vi "Config FX Set.vi"(5 "Max # Of Tries":i32, 6 "Send Cmd Timout(ms)":u32=300, 8 "Error":errorcluster, 9 "HW Config":T6={"LiftHW Ver"=0, "CAN"={"ID Primary"=0, "Bus"="", "ID Follower"=0}, "Output"={"Type"=enum."Counter-Clockwise", "Neutral"=enum."EEPROMSetting", "Max"={"FWD"=0.0, "REV"=-1.0}, "Min"={"FWD"=0.0, "REV"=0.0}, "OL Ramp Rate (S)"=0.0, "Dead Band"=0.0}, "CLUp"={"Gains"={"P"=1.0, "I"=0.01, "D"=0.0, "F"=0.0}, "Error Allowed"={"High"=0.0, "Low"=0.0}, "I Zone"={"High"=10000.0, "Low"=-1000.0}, "Max Out"={"FWD"=1.0, "REV"=-1.0}, "Max I Accu"={"High"=10.0, "Low"=-10.0}, "CL Ramp Rate (S)"=0.0}, "MM"={"Cruise Velocity"=5000, "Acceleration"=5000}, "TravelLimits"={"Hard"={"FWD Switch Normal"=enum."Normally Open", "FWD On will Zero Encoder "=FALSE, "REV Switch Normal"=enum."Normally Open", "REV On will Zero Encoder "=FALSE}, "Soft"={"FWD"={"Enable"=FALSE, "Counts"=0}, "REV"={"Enable"=FALSE, "Counts"=0}}}, "Cancoder"={"ID"=0, "CW(t) CCW(f)"=TRUE, "Zero Offset"=0.0}, "CLDown"={"Gains"={"P"=1.0, "I"=0.01, "D"=0.0, "F"=0.0}, "Error Allowed"={"High"=0.0, "Low"=0.0}, "I Zone"={"High"=10000.0, "Low"=-1000.0}, "Max Out"={"FWD"=1.0, "REV"=-1.0}, "Max I Accu"={"High"=10.0, "Low"=-10.0}, "CL Ramp Rate (S)"=0.0}, "CurrentLimit"={"Enable"=FALSE, "Current Limit"=0.0, "Threshold Current"=0.0, "Threshold Time"=0.0}} {"CLDown"."Max I Accu"."Low" format="%#.8f"; "CLDown"."Max I Accu"."High" format="%#.8f"; "CLDown"."Gains"."F" format="%#.8f"; "CLDown"."Gains"."D" format="%#.8f"; "CLDown"."Gains"."I" format="%#.8f"; "CLDown"."Gains"."P" format="%#.8f"; "CLDown"."Error Allowed"."Low" format="%#.8f"; "CLDown"."Error Allowed"."High" format="%#.8f"; "CLDown"."I Zone"."Low" format="%#.8f"; "CLDown"."I Zone"."High" format="%#.8f"; "CLDown"."Max Out"."REV" format="%.2f"; "CLDown"."Max Out"."FWD" format="%.2f"; "TravelLimits"."Soft"."REV"."Counts" format="%#.0f"; "TravelLimits"."Soft"."FWD"."Counts" format="%#.0f"; "Output"."Min"."REV" format="%.2f"; "Output"."Min"."FWD" format="%.2f"; "Output"."Max"."REV" format="%.2f"; "Output"."Max"."FWD" format="%.2f"; "CLUp"."Max I Accu"."Low" format="%#.8f"; "CLUp"."Max I Accu"."High" format="%#.8f"; "CLUp"."Gains"."F" format="%#.8f"; "CLUp"."Gains"."D" format="%#.8f"; "CLUp"."Gains"."I" format="%#.8f"; "CLUp"."Gains"."P" format="%#.8f"; "CLUp"."Error Allowed"."Low" format="%#.8f"; "CLUp"."Error Allowed"."High" format="%#.8f"; "CLUp"."I Zone"."Low" format="%#.8f"; "CLUp"."I Zone"."High" format="%#.8f"; "CLUp"."Max Out"."REV" format="%.2f"; "CLUp"."Max Out"."FWD" format="%.2f"}, 11 "PhoenixMotorControlDevRef":T1={"DeviceStatus"={"status"=FALSE, "code"=0, "source"=""}, "Type"=enum."PWM", "PWM"={"PWM Channel"=enum."Invalid", "DeadBand"={"Name"="", "maxPositivePwm"=0, "minPositivePwm"=0, "centerPwm"=0, "maxNegativePwm"=0, "minNegativePwm"=0, "angularRange"=0}}, "CAN"={"Device Number"=0, "SetOutput VI Ref"=variant, "GetOutput VI Ref"=variant, "Enable VI Ref"=variant, "Disable VI Ref"=variant, "Data"=variant}, "Invert"=FALSE, "DIO PWM"={"PWM \"Enable\" Channel"=enum."Invalid", "DIOChannel"=enum."Invalid", "PWM Rate"=0.0}}) -> (0 "Error Out":errorcluster, 3 "PhoenixMotorControlDevRef Out Out":T1)   [LabVIEW 2023, in "Lift_ACT.lvlib"]
uses:
  Lift_ACT.lvlib
  <vilib>/Utility/Data Type/NI_Data Type.lvlib
  Shared Code/TypeDefs/Cluser_CAN Data.ctl
  <vilib>/Rock Robotics/WPI/ThirdParty/Phoenix-LabVIEW/Motor Controller/Controls/CTRE_Phoenix_MotorControl_TalonFXInvertType.ctl
  <vilib>/Rock Robotics/WPI/ThirdParty/Phoenix-LabVIEW/Motor Controller/Controls/CTRE_Phoenix_MotorControl_NeutralMode.ctl
  Shared Code/TypeDefs/Cluster_FWD  REV Values.ctl
  Shared Code/TypeDefs/Cluster_Config Motor Output.ctl
  Shared Code/TypeDefs/Cluster_PID Gains.ctl
  Shared Code/TypeDefs/Cluster_High-Low.ctl
  Shared Code/TypeDefs/Cluster_PID Config.ctl
  Shared Code/TypeDefs/Cluster_Motion Magic Parameters.ctl
  <vilib>/Rock Robotics/WPI/ThirdParty/Phoenix-LabVIEW/Motor Controller/Controls/CTRE_Phoenix_MotorControl_LimitSwitchNormal.ctl
  Shared Code/TypeDefs/Cluser_Hard Limits.ctl
  Shared Code/TypeDefs/Cluser_Enable-Value I32.ctl
  Shared Code/TypeDefs/Cluser_Config_Soft Limits.ctl
  Shared Code/TypeDefs/Cluser_Limit Travel Config.ctl
  <vilib>/Rock Robotics/WPI/ThirdParty/Phoenix-LabVIEW/Motor Controller/Controls/CTRE_Phoenix_MotorControl_RemoteSourceType.ctl
  <vilib>/Rock Robotics/WPI/ThirdParty/Phoenix-LabVIEW/Motor Controller/Controls/CTRE_Phoenix_MotorControl_FeedbackDevice_TalonFX.ctl
  Shared Code/TypeDefs/Cluster_Config FX Motor Output.ctl
  Shared Code/TypeDefs/Cluster_FX SLOT PID Config.ctl
  <vilib>/Rock Robotics/SystemInterfaces/DIO/FPGA_DIOPWMChannel.ctl
  <vilib>/Rock Robotics/WPI/PWM/WPI_PWMDeadband.ctl
  <vilib>/Rock Robotics/WPI/MotorControl/WPI_MotorControlType.ctl
  <vilib>/Rock Robotics/SystemInterfaces/DIO/FPGA_DIOChannel.ctl
  <vilib>/Rock Robotics/WPI/MotorControl/WPI_MotorControlDeviceRef.ctl
  Shared Code/TypeDefs/Cluster_Config_Cancoder Data.ctl
  Shared Code/TypeDefs/Cluster_Lift_Config HW Values.ctl
  Shared Code/TypeDefs/Cluser_CAN Follower Data.ctl
  Shared Code/TypeDefs/Cluser_Config_Current Limits.ctl
panel:
  # "Tune Output\nto 1023 Max"
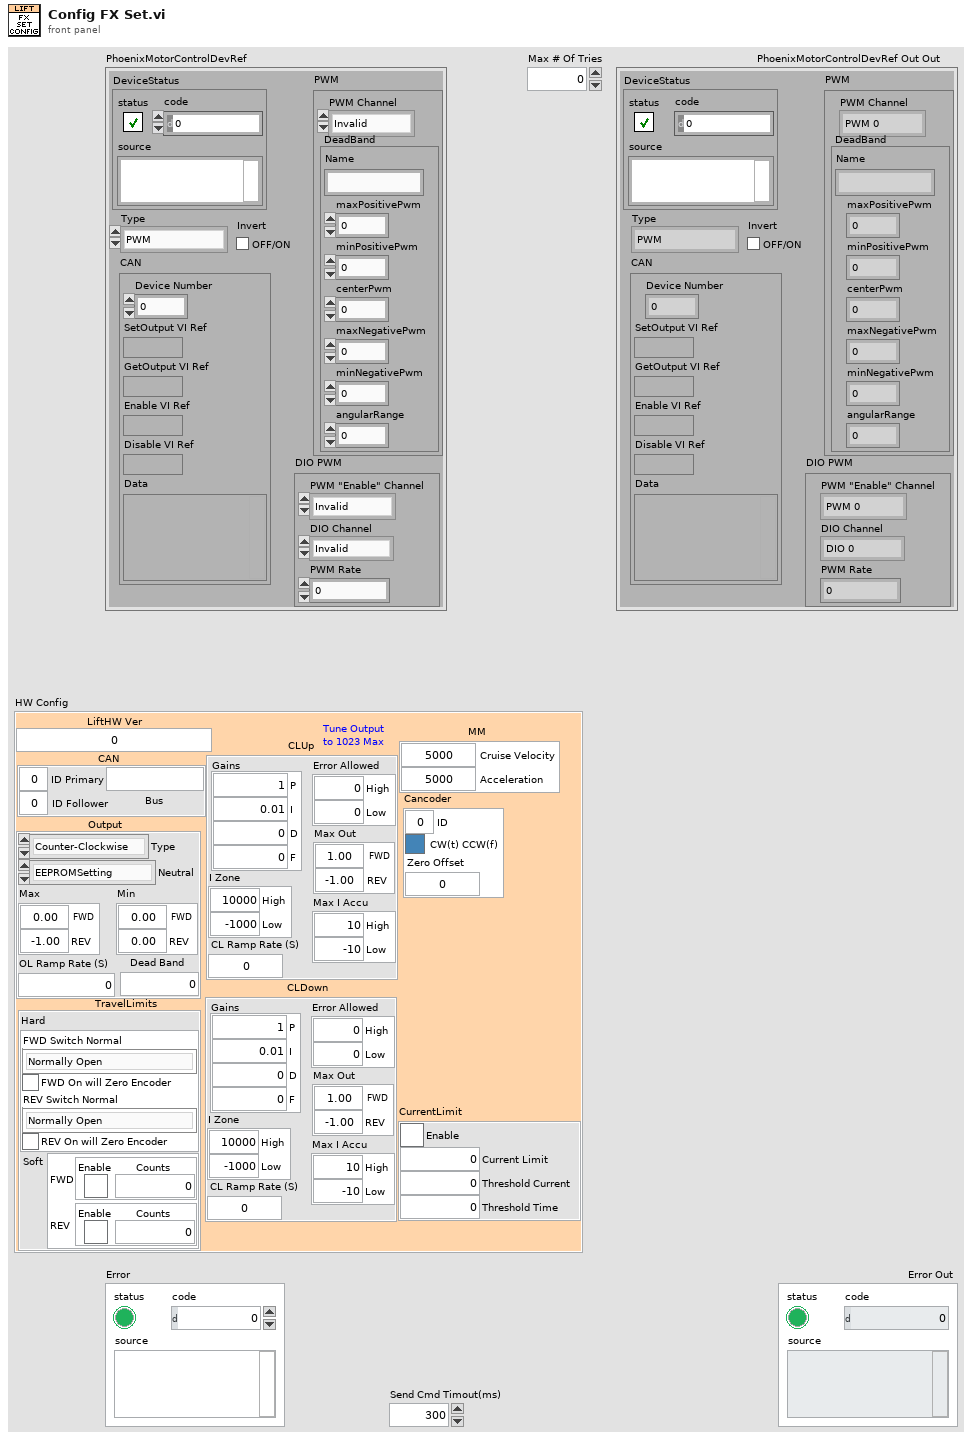
[diagram p1: front panel]
types:
  T1 = typedef "WPI_MotorControlDeviceRef.ctl" = cluster{"DeviceStatus":errorcluster, "Type":T2, "PWM":cluster{"PWM Channel":T3, "DeadBand":T4}, "CAN":cluster{"Device Number":u8, "SetOutput VI Ref":variant, "GetOutput VI Ref":variant, "Enable VI Ref":variant, "Disable VI Ref":variant, "Data":variant}, "Invert":bool, "DIO PWM":cluster{"PWM \"Enable\" Channel":T3, "DIOChannel":T5, "PWM Rate":dbl}}
  T2 = typedef "WPI_MotorControlType.ctl" = enum16{"PWM", "CAN", "DIO PWM"}
  T3 = typedef "FPGA_DIOPWMChannel.ctl" = enum8{"PWM 0", "PWM 1", "PWM 2", "PWM 3", "PWM 4", "PWM 5", "PWM 6", "PWM 7", "PWM 8", "PWM 9", "PWM MXP 0", "PWM MXP 1", "PWM MXP 2", "PWM MXP 3", "PWM MXP 4", "PWM MXP 5", "PWM MXP 6", "PWM MXP 7", "PWM MXP 8", "PWM MXP 9", "Invalid"}
  T4 = typedef "WPI_PWMDeadband.ctl" = cluster{"Name":string, "maxPositivePwm":i32, "minPositivePwm":i32, "centerPwm":i32, "maxNegativePwm":i32, "minNegativePwm":i32, "angularRange":u16}
  T5 = typedef "FPGA_DIOChannel.ctl" = enum8{"DIO 0", "DIO 1", "DIO 2", "DIO 3", "DIO 4", "DIO 5", "DIO 6", "DIO 7", "DIO 8", "DIO 9", "DIO MXP 0", "DIO MXP 1", "DIO MXP 2", "DIO MXP 3", "DIO MXP 4", "DIO MXP 5", "DIO MXP 6", "DIO MXP 7", "DIO MXP 8", "DIO MXP 9", "DIO MXP 10", "DIO MXP 11", "DIO MXP 12", "DIO MXP 13", "DIO MXP 14", "DIO MXP 15", "SPI Port CS1", "SPI Port CS2", "SPI Port CS3", "SPI Port MISO", "SPI Port MOSI", "Invalid"}
  T6 = typedef "Cluster_Lift_Config HW Values.ctl" = cluster{"LiftHW Ver":u64, "CAN":T7, "Output":T8, "CLUp":T12, "MM":T15, "TravelLimits":T16, "Cancoder":T21, "CLDown":T12, "CurrentLimit":T22}
  T7 = typedef "Cluser_CAN Follower Data.ctl" = cluster{"ID Primary":u8, "Bus":string, "ID Follower":u8}
  T8 = typedef "Cluster_Config Motor Output.ctl" = cluster{"Type":T9, "Neutral":T10, "Max":T11, "Min":T11, "OL Ramp Rate (S)":dbl, "Dead Band":dbl}
  T9 = typedef "CTRE_Phoenix_MotorControl_TalonFXInvertType.ctl" = enum16{"Counter-Clockwise", "Clockwise"}
  T10 = typedef "CTRE_Phoenix_MotorControl_NeutralMode.ctl" = enum8{"EEPROMSetting", "Override to Coast", "Override to Brake"}
  T11 = typedef "Cluster_FWD  REV Values.ctl" = cluster{"FWD":dbl, "REV":dbl}
  T12 = typedef "Cluster_PID Config.ctl" = cluster{"Gains":T13, "Error Allowed":T14, "I Zone":T14, "Max Out":T11, "Max I Accu":T14, "CL Ramp Rate (S)":dbl}
  T13 = typedef "Cluster_PID Gains.ctl" = cluster{"P":dbl, "I":dbl, "D":dbl, "F":dbl}
  T14 = typedef "Cluster_High-Low.ctl" = cluster{"High":dbl, "Low":dbl}
  T15 = typedef "Cluster_Motion Magic Parameters.ctl" = cluster{"Cruise Velocity":i32, "Acceleration":i32}
  T16 = typedef "Cluser_Limit Travel Config.ctl" = cluster{"Hard":T17, "Soft":T19}
  T17 = typedef "Cluser_Hard Limits.ctl" = cluster{"FWD Switch Normal":T18, "FWD On will Zero Encoder ":bool, "REV Switch Normal":T18, "REV On will Zero Encoder ":bool}
  T18 = typedef "CTRE_Phoenix_MotorControl_LimitSwitchNormal.ctl" = enum16{"Normally Open", "Normally Closed", "Disabled"}
  T19 = typedef "Cluser_Config_Soft Limits.ctl" = cluster{"FWD":T20, "REV":T20}
  T20 = typedef "Cluser_Enable-Value I32.ctl" = cluster{"Enable":bool, "Counts":i32}
  T21 = typedef "Cluster_Config_Cancoder Data.ctl" = cluster{"ID":u8, "CW(t) CCW(f)":bool, "Zero Offset":dbl}
  T22 = typedef "Cluser_Config_Current Limits.ctl" = cluster{"Enable":bool, "Current Limit":dbl, "Threshold Current":dbl, "Threshold Time":dbl}
  T23 = typedef "Cluser_CAN Data.ctl" = cluster{"ID":u8, "Bus":string}
  T24 = enum16{"FollowerType_PercentOutput", "FollowerType_AuxOutput1"}
  T25 = typedef "Cluster_FX SLOT PID Config.ctl" = cluster{"Gains":T13, "Error Allowed":dbl, "I Zone":dbl, "Peak Out 0-1":dbl, "Max I Accu":dbl}
  T26 = typedef "Cluster_Config FX Motor Output.ctl" = cluster{"Type":T9, "Neutral":T10, "Max":T11, "Min":T11, "OL Ramp Rate (S)":dbl, "Dead Band":dbl, "CL Ramp Rate (S)":dbl}
  T27 = typedef "CTRE_Phoenix_MotorControl_RemoteSourceType.ctl" = enum16{"Off", "Talon SRX Selected Sensor", "Pigeon IMU Yaw", "Pigeon IMU Pitch", "Pigeon IMU Roll", "CANifier Quadrature", "CANifier PWM Input 0", "CANifier PWM Input 1", "CANifier PWM Input 2", "CANifier PWM Input 3", "Gadgeteer Pigeon Yaw", "Gadgeteer Pigeon Pitch", "Gadgeteer Pigeon Roll", "CANCoder"}
  T28 = typedef "CTRE_Phoenix_MotorControl_FeedbackDevice_TalonFX.ctl" = i8
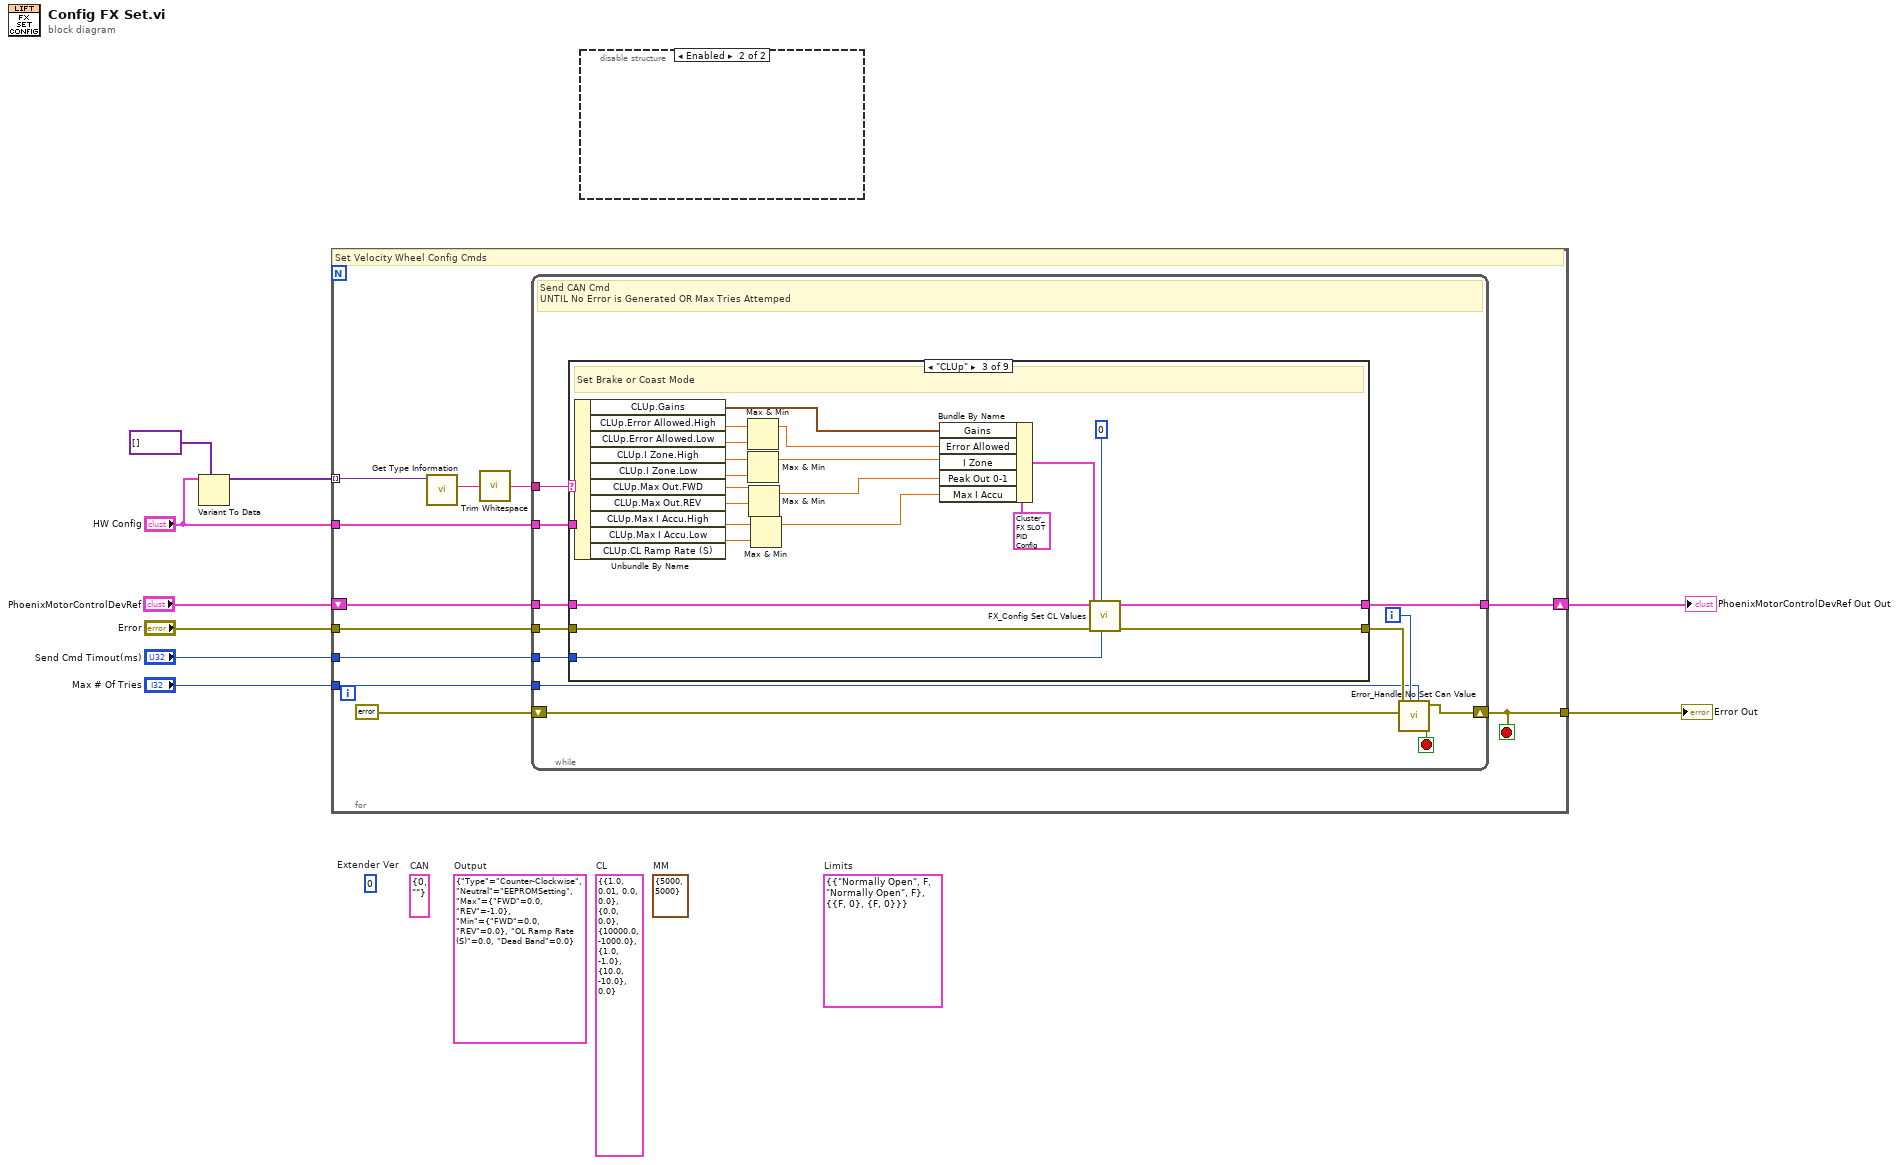
[diagram p0: block diagram]
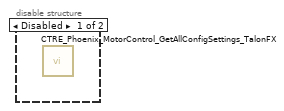
[diagram p2: hidden frame]
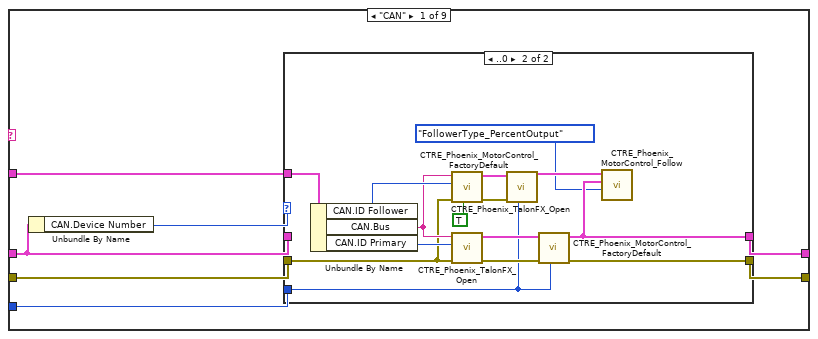
[diagram p3: hidden frame]
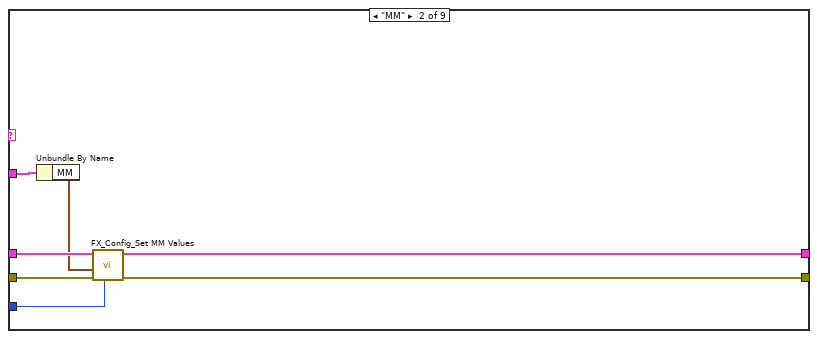
[diagram p5: hidden frame]
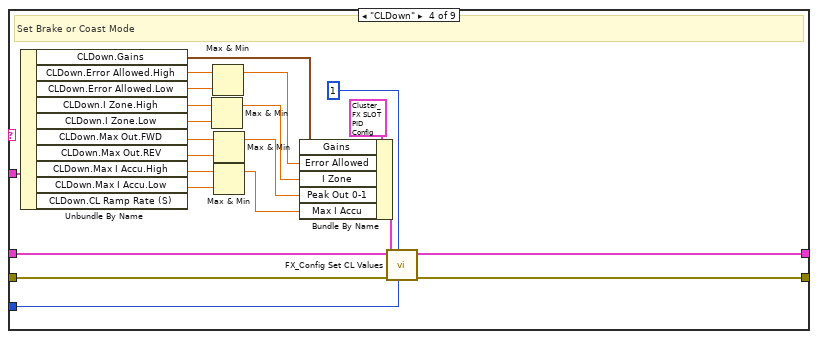
[diagram p6: hidden frame]
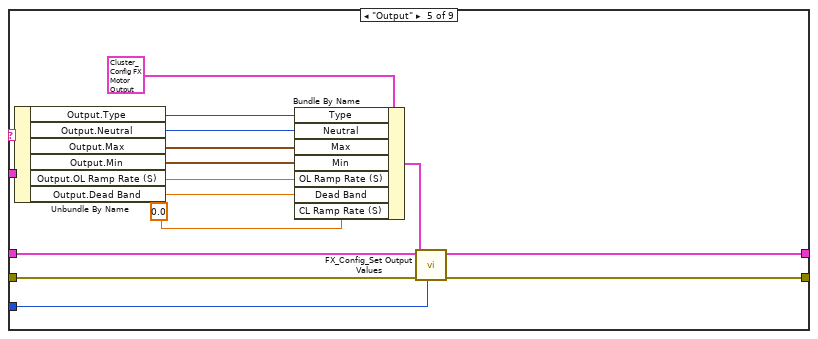
[diagram p7: hidden frame]
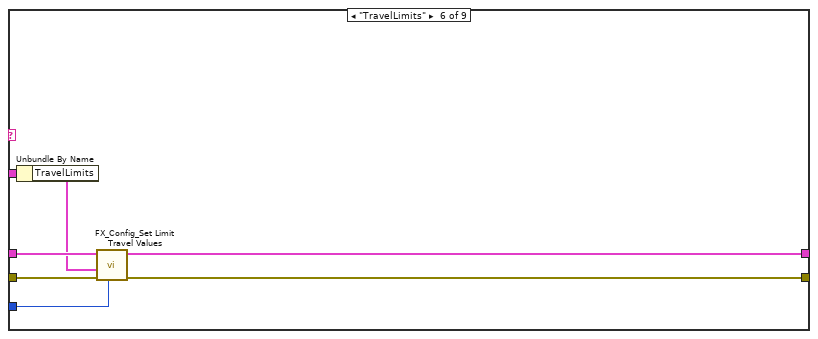
[diagram p8: hidden frame]
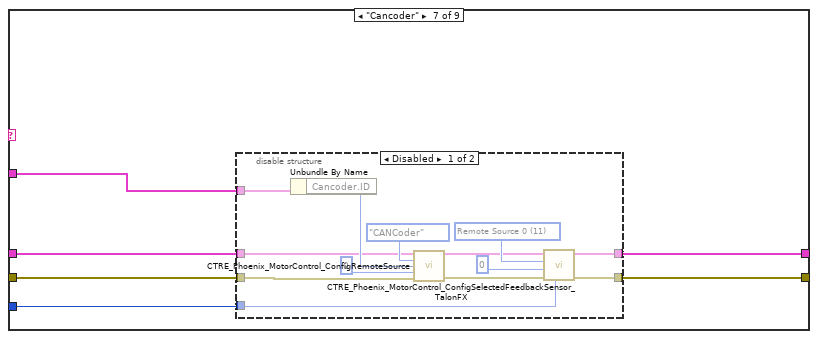
[diagram p9: hidden frame]
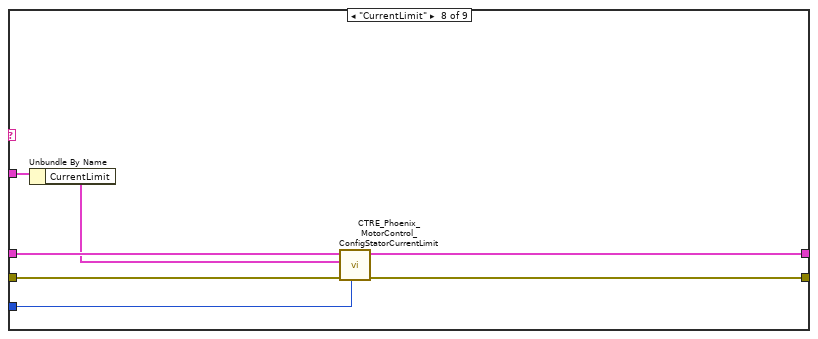
[diagram p11: hidden frame]
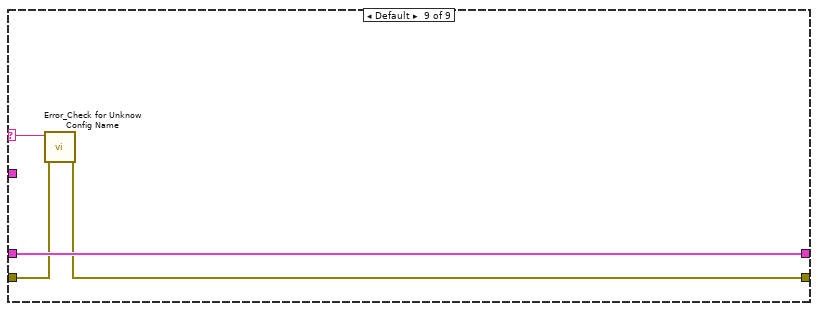
[diagram p12: hidden frame]
diagram:
  (unwired) T16 {"Hard"={"FWD Switch Normal"=enum."Normally Open", "FWD On will Zero Encoder "=FALSE, "REV Switch Normal"=enum."Normally Open", "REV On will Zero Encoder "=FALSE}, "Soft"={"FWD"={"Enable"=FALSE, "Counts"=0}, "REV"={"Enable"=FALSE, "Counts"=0}}}  # Limits
  (unwired) T15 {"Cruise Velocity"=5000, "Acceleration"=5000}  # MM
  (unwired) T12 {"Gains"={"P"=1.0, "I"=0.01, "D"=0.0, "F"=0.0}, "Error Allowed"={"High"=0.0, "Low"=0.0}, "I Zone"={"High"=10000.0, "Low"=-1000.0}, "Max Out"={"FWD"=1.0, "REV"=-1.0}, "Max I Accu"={"High"=10.0, "Low"=-10.0}, "CL Ramp Rate (S)"=0.0}  # CL
  (unwired) T8 {"Type"=enum."Counter-Clockwise", "Neutral"=enum."EEPROMSetting", "Max"={"FWD"=0.0, "REV"=-1.0}, "Min"={"FWD"=0.0, "REV"=0.0}, "OL Ramp Rate (S)"=0.0, "Dead Band"=0.0}  # Output
  (unwired) T23 {"ID"=0, "Bus"=""}  # CAN
  (unwired) u64 0  # Extender Ver
  n1 = Variant To Data(type=variant[] [] ("appended array"), Variant="HW Config") -> (data=w1:variant[])  [unwired: 1 in, 1 out]
  n2 = for {
    tunnel: "Send Cmd Timout(ms)" -> [w19]
    shift-right: [w20] -> w6
    shift-left: "PhoenixMotorControlDevRef" -> [w17]
    tunnel: "HW Config" -> [w18]
    tunnel: "Max # Of Tries" -> [w15]
    tunnel: w1 -> [w14] mode=indexing
    tunnel: "Error" -> [w16]
    tunnel: [w13] -> w5
    stop <- w13 stop-if-true
    # "Set Velocity Wheel Config Cmds"
    n3 = call <vilib>:"Get Type Information.vi"("variant"=w14) -> ("name"=w11:string)  [unwired: 6 in, 4 out]
    n4 = call <vilib>:"Trim Whitespace.vi"("string"=w11) -> ("trimmed string"=w10:string)  [unwired: 1 in]
    n5 = while {
      tunnel: [w24] -> w20
      tunnel: w19 -> [w30]
      shift-right: [w31] -> w13
      shift-left: errorcluster {"status"=FALSE, "code"=0, "source"=""} ("Error Out") -> [w29]
      tunnel: w16 -> [w27]
      tunnel: w17 -> [w26]
      tunnel: w18 -> [w25]
      tunnel: w15 -> [w23]
      tunnel: w10 -> [w22]
      i -> [w28]
      stop <- w21 stop-if-true
      # "Send CAN Cmd\nUNTIL No Error is Generated OR Max Tries Attemped"
      n6 = case shown="\"CLUp\"" w22 {
        selector: w22 -> [_ _ _ _ _ _ _ _ w160]
        tunnel: [w39 w62 w83 w105 w120 w127 w135 w157 w158] -> w32
        tunnel: w30 -> [w37 w61 w79 w101 w118 w125 w133 w155 _]
        tunnel: w27 -> [w38 w63 w82 w104 w119 w126 w134 w156 w159]
        tunnel: w26 -> [w35 w60 w85 w107 w121 w128 w132 w153 w161]
        tunnel: w25 -> [w33 w59 w81 w103 w117 w124 w130 w152 _]
        tunnel: [w34 w58 w84 w106 w122 w129 w131 w154 w161] -> w24
        frame "CAN" {
          n7 = Unbundle By Name(w35) -> ("CAN.Device Number"=w36:u8)
          n8 = case shown="..0" w36 {
            tunnel: [w40 w53] -> w39
            tunnel: w38 -> [w40 w46]
            tunnel: w37 -> [_ w49]
            tunnel: w35 -> [w41 _]
            tunnel: [w41 w44] -> w34
            tunnel: w33 -> [_ w52]
            frame 1.. {
            }
            frame ..0 {
              n9 = Unbundle By Name(w52) -> ("CAN.ID Follower"=w51:u8, "CAN.Bus"=w47:string, "CAN.ID Primary"=w54:u8)
              n10 = call <vilib>:"CTRE_Phoenix_TalonFX_Open.vi"("Invert"=TRUE, "error in"=w46, "Device Number"=w51, "CAN Bus"=w47) -> ("error out"=w48:errorcluster, "PhoenixMotorControlDevRef"=w50:T1)  [unwired: 6 in]
              n11 = call <vilib>:"CTRE_Phoenix_TalonFX_Open.vi"("error in"=w46, "Device Number"=w54, "CAN Bus"=w47) -> ("error out"=w55:errorcluster, "PhoenixMotorControlDevRef"=w56:T1)  [unwired: 7 in]
              n12 = call <vilib>:"CTRE_Phoenix_MotorControl_FactoryDefault.vi"("timeoutMs"=w49, "error in"=w48, "PhoenixMotorControlDevRef"=w50) -> ("PhoenixMotorControlDevRef"=w45:T1)  [unwired: 7 in, 1 out]
              n13 = call <vilib>:"CTRE_Phoenix_MotorControl_FactoryDefault.vi"("timeoutMs"=w49, "error in"=w55, "PhoenixMotorControlDevRef"=w56) -> ("error out"=w53:errorcluster, "PhoenixMotorControlDevRef"=w44:T1)  [unwired: 7 in]
              n14 = call <vilib>:"CTRE_Phoenix_MotorControl_Follow.vi"("FollowerType"=T24."FollowerType_PercentOutput", "Master Controller to Follow"=w44, "PhoenixMotorControlDevRef"=w45) -> ()  [unwired: 7 in, 2 out]
            }
          }
        }
        frame "MM" {
          n15 = Unbundle By Name(w59) -> ("MM"=w57:T15)
          n16 = call "FX_Config_Set MM Values.vi"("Send Cmd Timout(ms)"=w61, "Error"=w63, "MM"=w57, "PhoenixMotorControlDevRef"=w60) -> ("Error Out"=w62:errorcluster, "PhoenixMotorControlDevRef Out"=w58:T1)  [unwired: 6 in]
        }
        frame "CLUp" {
          # "Set Brake or Coast Mode"
          n17 = Unbundle By Name(w81) -> ("CLUp.Gains"=w76:T13, "CLUp.Error Allowed.High"=w75:dbl, "CLUp.Error Allowed.Low"=w74:dbl, "CLUp.I Zone.High"=w71:dbl, "CLUp.I Zone.Low"=w72:dbl, "CLUp.Max Out.FWD"=w69:dbl, "CLUp.Max Out.REV"=w68:dbl, "CLUp.Max I Accu.High"=w66:dbl, "CLUp.Max I Accu.Low"=w65:dbl)  [unwired: 1 out]
          n18 = Max & Min(x=w75, y=w74) -> (max(x,y)=w73:dbl)  [unwired: 1 out]
          n19 = Max & Min(x=w71, y=w72) -> (max(x,y)=w70:dbl)  [unwired: 1 out]
          n20 = Max & Min(x=w69, y=w68) -> (max(x,y)=w67:dbl)  [unwired: 1 out]
          n21 = Max & Min(x=w66, y=w65) -> (max(x,y)=w64:dbl)  [unwired: 1 out]
          n22 = Bundle By Name(cluster=T25 {"Gains"={"P"=0.0, "I"=0.0, "D"=0.0, "F"=0.0}, "Error Allowed"=0.0, "I Zone"=0.0, "Peak Out 0-1"=0.0, "Max I Accu"=0.0} ("CL"), "Gains"=w76, "Error Allowed"=w73, "I Zone"=w70, "Peak Out 0-1"=w67, "Max I Accu"=w64) -> (w77:T25)
          n23 = call "FX_Config Set CL Values.vi"("Send Cmd Timout(ms)"=w79, "SlotIdx"=0, "Error"=w82, "CL"=w77, "PhoenixMotorControlDevRef"=w85) -> ("Error Out"=w83:errorcluster, "PhoenixMotorControlDevRef Out"=w84:T1)  [unwired: 4 in, 1 out]
        }
        frame "CLDown" {
          # "Set Brake or Coast Mode"
          n24 = Unbundle By Name(w103) -> ("CLDown.Gains"=w96:T13, "CLDown.Error Allowed.High"=w97:dbl, "CLDown.Error Allowed.Low"=w98:dbl, "CLDown.I Zone.High"=w94:dbl, "CLDown.I Zone.Low"=w93:dbl, "CLDown.Max Out.FWD"=w90:dbl, "CLDown.Max Out.REV"=w91:dbl, "CLDown.Max I Accu.High"=w88:dbl, "CLDown.Max I Accu.Low"=w87:dbl)  [unwired: 1 out]
          n25 = Max & Min(x=w94, y=w93) -> (max(x,y)=w92:dbl)  [unwired: 1 out]
          n26 = Max & Min(x=w97, y=w98) -> (max(x,y)=w95:dbl)  [unwired: 1 out]
          n27 = Max & Min(x=w90, y=w91) -> (max(x,y)=w89:dbl)  [unwired: 1 out]
          n28 = Max & Min(x=w88, y=w87) -> (max(x,y)=w86:dbl)  [unwired: 1 out]
          n29 = Bundle By Name(cluster=T25 {"Gains"={"P"=0.0, "I"=0.0, "D"=0.0, "F"=0.0}, "Error Allowed"=0.0, "I Zone"=0.0, "Peak Out 0-1"=0.0, "Max I Accu"=0.0} ("CL"), "Gains"=w96, "Error Allowed"=w95, "I Zone"=w92, "Peak Out 0-1"=w89, "Max I Accu"=w86) -> (w99:T25)
          n30 = call "FX_Config Set CL Values.vi"("Send Cmd Timout(ms)"=w101, "SlotIdx"=1, "Error"=w104, "CL"=w99, "PhoenixMotorControlDevRef"=w107) -> ("Error Out"=w105:errorcluster, "PhoenixMotorControlDevRef Out"=w106:T1)  [unwired: 4 in, 1 out]
        }
        frame "Output" {
          n31 = Unbundle By Name(w117) -> ("Output.Type"=w108:T9, "Output.Neutral"=w109:T10, "Output.Max"=w110:T11, "Output.Min"=w111:T11, "Output.OL Ramp Rate (S)"=w112:dbl, "Output.Dead Band"=w113:dbl)
          n32 = Bundle By Name(cluster=T26 {"Type"=enum."Counter-Clockwise", "Neutral"=enum."EEPROMSetting", "Max"={"FWD"=0.0, "REV"=0.0}, "Min"={"FWD"=0.0, "REV"=0.0}, "OL Ramp Rate (S)"=0.0, "Dead Band"=0.0, "CL Ramp Rate (S)"=0.0} ("Output"), "Type"=w108, "Neutral"=w109, "Max"=w110, "Min"=w111, "OL Ramp Rate (S)"=w112, "Dead Band"=w113, "CL Ramp Rate (S)"=0.0) -> (w115:T26)
          n33 = call "FX_Config_Set Output Values.vi"("Send Cmd Timout(ms)"=w118, "Error"=w119, "Output"=w115, "PhoenixMotorControlDevRef"=w121) -> ("Error Out"=w120:errorcluster, "PhoenixMotorControlDevRef Out"=w122:T1)  [unwired: 6 in]
        }
        frame "TravelLimits" {
          n34 = Unbundle By Name(w124) -> ("TravelLimits"=w123:T16)
          n35 = call "FX_Config_Set Limit Travel Values.vi"("Send Cmd Timout(ms)"=w125, "Error"=w126, "Limits"=w123, "PhoenixMotorControlDevRef"=w128) -> ("Error Out"=w127:errorcluster, "PhoenixMotorControlDevRef Out"=w129:T1)  [unwired: 6 in]
        }
        frame "Cancoder" {
          n36 = disable-structure shown="Disabled" {
            disable-tunnel: [w141 w149] -> w135
            disable-tunnel: w134 -> [w140 w149]
            disable-tunnel: w133 -> [w139 _]
            disable-tunnel: w132 -> [w138 w150]
            disable-tunnel: [w137 w150] -> w131
            disable-tunnel: w130 -> [w136 _]
            frame Disabled {
              w145 = T28 11 items=["Integrated Sensor"=1, "Sensor Sum (S0 + S1)"=9, "Sensor Difference (D0 - D1)"=10, "Remote Source 0"=11, "Remote Source 1"=12, "None"=14, "Software Emulated"=15] ("Talon FX Feedback Device")
              n37 = Unbundle By Name(w136) -> ("Cancoder.ID"=w146:u8)
              n38 = call <vilib>:"CTRE_Phoenix_MotorControl_ConfigRemoteSource.vi"("PhoenixMotorControlDevRef"=w138, "Remote Device Type"=CTRE_Phoenix_MotorControl_RemoteSourceType."CANCoder", "Remote Device ID"=w146, "Source Index (0/1)"=u32 0, "error in (no error)"=w140) -> ("PhoenixMotorControlDevRef"=w142:T1, "error out"=w143:errorcluster)  [unwired: 9 in]
              n39 = call <vilib>:"CTRE_Phoenix_MotorControl_ConfigSelectedFeedbackSensor_TalonFX.vi"("timeoutMs"=w139, "error in (no error)"=w143, "pidLoopIdx"=0, "Talon FX Feedback Device"=w145, "PhoenixMotorControlDevRef"=w142) -> ("error out"=w141:errorcluster, "PhoenixMotorControlDevRef"=w137:T1)  [unwired: 5 in]
            }
            frame Enabled {
            }
          }
        }
        frame "CurrentLimit" {
          n40 = Unbundle By Name(w152) -> ("CurrentLimit"=w151:T22)
          n41 = call <vilib>:"CTRE_Phoenix_MotorControl_ConfigStatorCurrentLimit.vi"("timeoutMs"=w155, "error in (no error)"=w156, "Stator Current Limit Configuration"=w151, "PhoenixMotorControlDevRef"=w153) -> ("error out"=w157:errorcluster, "PhoenixMotorControlDevRef"=w154:T1)  [unwired: 6 in]
        }
        frame Default {
          n42 = call "Error_Check for Unknow Config Name.vi"("error in (no error)"=w159, "Config Name"=w160) -> ("error out"=w158:errorcluster)  [unwired: 9 in]
        }
      }
      n43 = call "Error_Handle No Set Can Value.vi"("Max # Of Tries"=w23, "Loop Itteration"=w28, "Previous Error"=w29, "Error"=w32) -> ("Stop Out"=w21:bool, "Error Out"=w31:errorcluster)  [unwired: 6 in]
    }
  }
  "Error Out" <- w5
  "PhoenixMotorControlDevRef Out Out" <- w6
  n44 = disable-structure shown="Enabled" {
    frame Disabled {
      n45 = call <vilib>:"CTRE_Phoenix_MotorControl_GetAllConfigSettings_TalonFX.vi"() -> ()  [unwired: 9 in, 3 out]
    }
    frame Enabled {
    }
  }
